vi "Obtain Message Queue.vi"(8 "error in (no error)":errorcluster) -> (0 "error out":errorcluster, 3 "Message Queue":refnum<queue>)   [LabVIEW 2020, in "Message Queue.lvlib"]
doc: "Create a queue with the Message Cluster data type."
uses:
  Message Queue.lvlib
  Message Cluster.ctl
  States.ctl
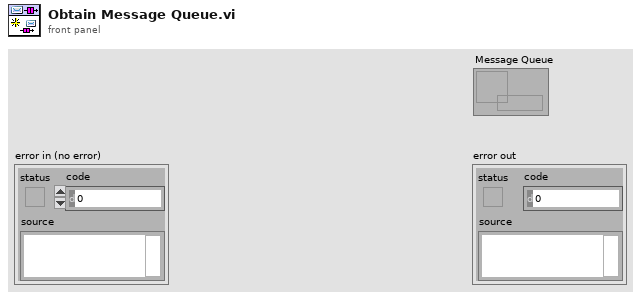
[diagram p1: front panel]
types:
  T1 = typedef "Message Queue.lvlib/Message Cluster.ctl" = cluster{"Message":T2, "Message Data":variant}
  T2 = typedef "Message Queue.lvlib/States.ctl" = enum16{"Init", "Update Display", "Assign Instruments", "Configure Evironmental", "Configure Device", "Update device info", "Calibrate Path", "Configure Test", "Init XML", "Init Environmental", "Next Environmental", "Run Tests", "Cancel Tests", "Change Data Path", "Update test list", "Finish test", "Exit", "Error", "Menu Selection"}
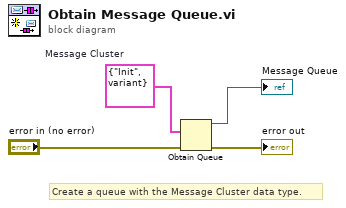
[diagram p0: block diagram]
diagram:
  w4 = T1 {"Message"=enum."Init", "Message Data"=variant}  # Message Cluster
  # "Create a queue with the Message Cluster data type."
  n1 = Obtain Queue(element data type=w4, error in (no error)="error in (no error)") -> (queue out=→"Message Queue":refnum<queue>, error out=→"error out":errorcluster)  [unwired: 3 in, 1 out]
